vi "Launch Console.vi"() -> ()   [LabVIEW 2026]
panel:
  in  "Launch Button":bool
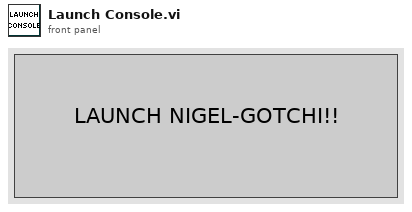
[diagram p1: front panel]
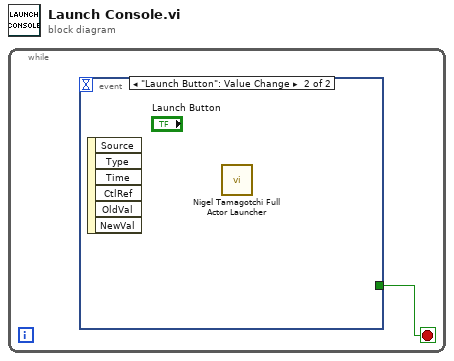
[diagram p0: block diagram]
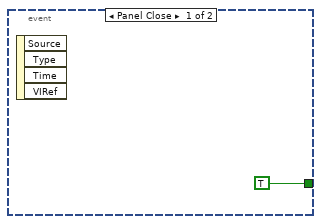
[diagram p2: hidden frame]
diagram:
  n1 = while {
    stop <- w1 stop-if-true
    n2 = event shown="[1] \"Launch Button\": Value Change" {
      selector: _ -> [_ _]
      dyn-events: _ -> [_ _]
      timeout: _ -> [_ _]
      tunnel: [TRUE _] -> w1
      event Panel Close {
        n3 = event-data() -> ()  [unwired: 1 in, 4 out]
      }
      event "Launch Button": Value Change {
        n4 = event-data() -> ()  [unwired: 1 in, 6 out]
        n5 = call "Nigel Tamagotchi Full Actor Launcher.vi"() -> ()  [unwired: 12 in]
      }
    }
  }
